vi "usrp rx info free.vi"(0 "rx_info":T1, 11 "error in (no error)":errorcluster) -> (1 "rx_antenna":string, 2 "rx_subdev_spec":string, 3 "rx_id":string, 4 "rx_info out":T1, 6 "mboard_id":string, 8 "mboard_name":string, 10 "mboard_serial":string, 12 "function return":u32(ring), 13 "rx_serial":string, 14 "rx_subdev_name":string, 15 "error out":errorcluster)   [LabVIEW 2023, in "uhd.lvlib"]
doc: "UHD_API uhd_error uhd_usrp_rx_info_free(uhd_usrp_rx_info_t* rx_info);"
uses:
  <vilib>/Utility/importsl/GetValueByPointer/datatype.ctl
  <vilib>/Utility/importsl/GetValueByPointer/GetValueByPointer.xnode
  <userlib>/uhd/uhd.lvlib
  <userlib>/uhd/uhd.dll
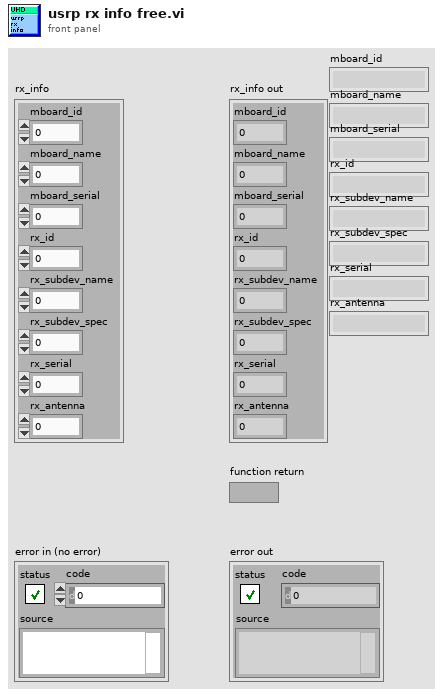
[diagram p1: front panel]
types:
  T1 = cluster{"mboard_id":u64, "mboard_name":u64, "mboard_serial":u64, "rx_id":u64, "rx_subdev_name":u64, "rx_subdev_spec":u64, "rx_serial":u64, "rx_antenna":u64}
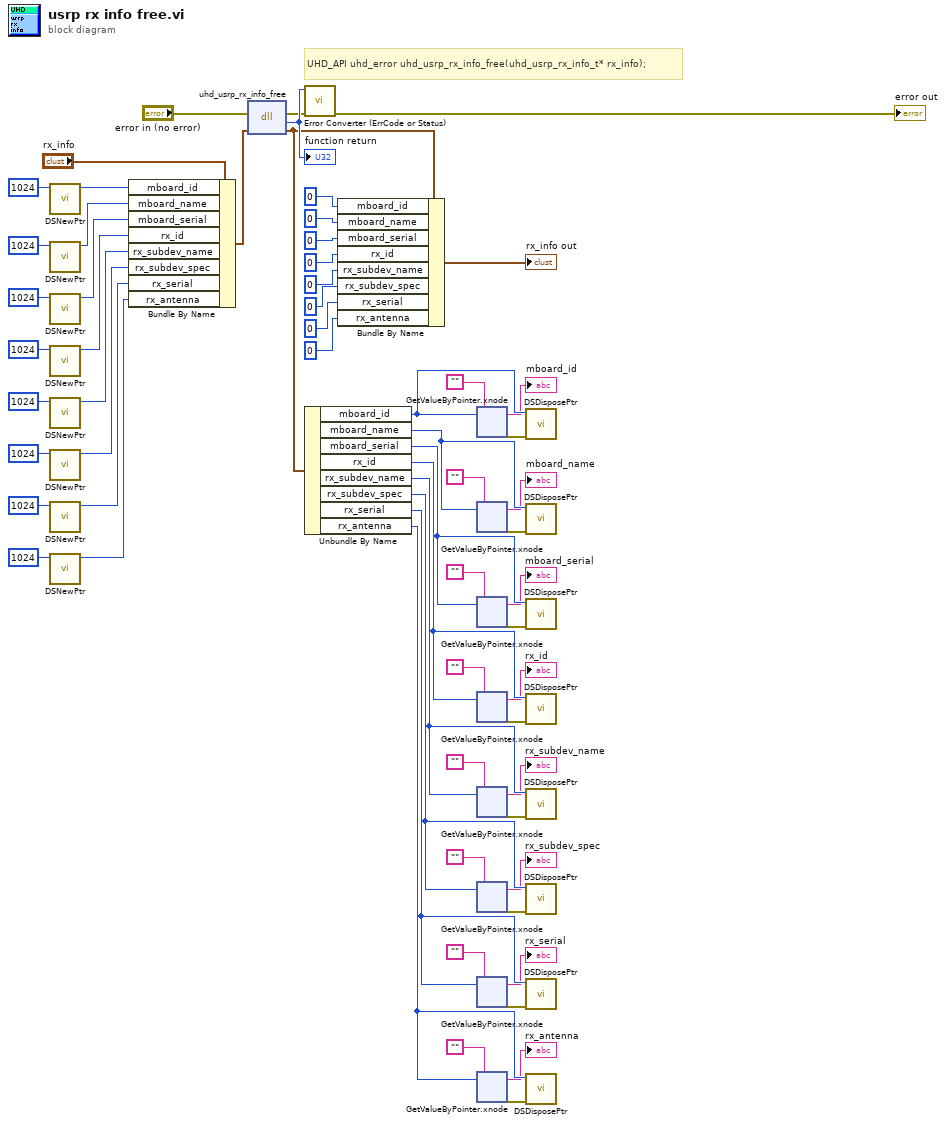
[diagram p0: block diagram]
diagram:
  # "UHD_API uhd_error uhd_usrp_rx_info_free(uhd_usrp_rx_info_t* rx_info);"
  n1 = call <vilib>:"DSNewPtr.vi"("Size"=u64 1024) -> ("Pointer"=w54:u64)  [unwired: 9 in, 1 out]
  n2 = call <vilib>:"DSNewPtr.vi"("Size"=u64 1024) -> ("Pointer"=w52:u64)  [unwired: 9 in, 1 out]
  n3 = call <vilib>:"DSNewPtr.vi"("Size"=u64 1024) -> ("Pointer"=w51:u64)  [unwired: 9 in, 1 out]
  n4 = call <vilib>:"DSNewPtr.vi"("Size"=u64 1024) -> ("Pointer"=w50:u64)  [unwired: 9 in, 1 out]
  n5 = call <vilib>:"DSNewPtr.vi"("Size"=u64 1024) -> ("Pointer"=w49:u64)  [unwired: 9 in, 1 out]
  n6 = call <vilib>:"DSNewPtr.vi"("Size"=u64 1024) -> ("Pointer"=w48:u64)  [unwired: 9 in, 1 out]
  n7 = call <vilib>:"DSNewPtr.vi"("Size"=u64 1024) -> ("Pointer"=w47:u64)  [unwired: 9 in, 1 out]
  n8 = call <vilib>:"DSNewPtr.vi"("Size"=u64 1024) -> ("Pointer"=w46:u64)  [unwired: 9 in, 1 out]
  n9 = Bundle By Name(cluster="rx_info", "mboard_id"=w54, "mboard_name"=w52, "mboard_serial"=w51, "rx_id"=w50, "rx_subdev_name"=w49, "rx_subdev_spec"=w48, "rx_serial"=w47, "rx_antenna"=w46) -> (w53:T1)
  n10 = dll-call lib="C:/Program Files/National Instruments/LabVIEW 2023/user.lib/uhd/uhd.*" fn="uhd_usrp_rx_info_free"(error in="error in (no error)", "rx_info"=w53) -> (error out=w2:errorcluster, w64:u32, "rx_info"=w13:T1)  [unwired: 2 in, 1 out]
  "function return" <- w64
  n11 = call <userlib>:"Error Converter (ErrCode or Status).vi"("error in (no error)"=w2, "error code"=w64) -> ("error out"=→"error out":errorcluster)  [unwired: 9 in]
  n12 = Unbundle By Name(w13) -> ("mboard_id"=w44:u64, "mboard_name"=w40:u64, "mboard_serial"=w36:u64, "rx_id"=w32:u64, "rx_subdev_name"=w28:u64, "rx_subdev_spec"=w24:u64, "rx_serial"=w20:u64, "rx_antenna"=w16:u64)
  n13 = Bundle By Name(cluster=w13, "mboard_id"=u64 0, "mboard_name"=u64 0, "mboard_serial"=u64 0, "rx_id"=u64 0, "rx_subdev_name"=u64 0, "rx_subdev_spec"=u64 0, "rx_serial"=u64 0, "rx_antenna"=u64 0) -> (→"rx_info out":T1)
  n14 = xnode "GetValueByPointer.xnode"("Pointer"=w44, "InputType"="") -> ("Output"=→"mboard_id":string, "ErrorOut"=w45:errorcluster)  [unwired: 2 in]
  n15 = xnode "GetValueByPointer.xnode"("Pointer"=w40, "InputType"="") -> ("Output"=→"mboard_name":string, "ErrorOut"=w41:errorcluster)  [unwired: 2 in]
  n16 = xnode "GetValueByPointer.xnode"("Pointer"=w36, "InputType"="") -> ("Output"=→"mboard_serial":string, "ErrorOut"=w37:errorcluster)  [unwired: 2 in]
  n17 = xnode "GetValueByPointer.xnode"("Pointer"=w32, "InputType"="") -> ("Output"=→"rx_id":string, "ErrorOut"=w33:errorcluster)  [unwired: 2 in]
  n18 = xnode "GetValueByPointer.xnode"("Pointer"=w28, "InputType"="") -> ("Output"=→"rx_subdev_name":string, "ErrorOut"=w29:errorcluster)  [unwired: 2 in]
  n19 = xnode "GetValueByPointer.xnode"("Pointer"=w24, "InputType"="") -> ("Output"=→"rx_subdev_spec":string, "ErrorOut"=w25:errorcluster)  [unwired: 2 in]
  n20 = xnode "GetValueByPointer.xnode"("Pointer"=w20, "InputType"="") -> ("Output"=→"rx_serial":string, "ErrorOut"=w21:errorcluster)  [unwired: 2 in]
  n21 = xnode "GetValueByPointer.xnode"("Pointer"=w16, "InputType"="") -> ("Output"=→"rx_antenna":string, "ErrorOut"=w17:errorcluster)  [unwired: 2 in]
  n22 = call <vilib>:"DSDisposePtr.vi"("error in (no error)"=w45, "Pointer"=w44) -> ()  [unwired: 9 in, 1 out]
  n23 = call <vilib>:"DSDisposePtr.vi"("error in (no error)"=w41, "Pointer"=w40) -> ()  [unwired: 9 in, 1 out]
  n24 = call <vilib>:"DSDisposePtr.vi"("error in (no error)"=w37, "Pointer"=w36) -> ()  [unwired: 9 in, 1 out]
  n25 = call <vilib>:"DSDisposePtr.vi"("error in (no error)"=w33, "Pointer"=w32) -> ()  [unwired: 9 in, 1 out]
  n26 = call <vilib>:"DSDisposePtr.vi"("error in (no error)"=w29, "Pointer"=w28) -> ()  [unwired: 9 in, 1 out]
  n27 = call <vilib>:"DSDisposePtr.vi"("error in (no error)"=w25, "Pointer"=w24) -> ()  [unwired: 9 in, 1 out]
  n28 = call <vilib>:"DSDisposePtr.vi"("error in (no error)"=w21, "Pointer"=w20) -> ()  [unwired: 9 in, 1 out]
  n29 = call <vilib>:"DSDisposePtr.vi"("error in (no error)"=w17, "Pointer"=w16) -> ()  [unwired: 9 in, 1 out]
